vi "Read Track.vi"(7 "Track Controls":T1 {"Track 3"."Volume Settings"."Volume" scale=1.0..10.0; "Track 3"."Volume Settings"."Pan" scale=0.0..1.0; "Track 3"."Effects Settings"."Delay 2" scale=0.0..10.0; "Track 3"."Effects Settings"."Delay" scale=0.0..1.0; "Track 2"."Volume Settings"."Volume" scale=1.0..10.0; "Track 2"."Volume Settings"."Pan" scale=0.0..1.0; "Track 2"."Effects Settings"."Delay 2" scale=0.0..10.0; "Track 2"."Effects Settings"."Delay" scale=0.0..1.0; "Track 1"."Volume Settings"."Volume" scale=1.0..10.0; "Track 1"."Volume Settings"."Pan" scale=0.0..1.0; "Track 1"."Effects Settings"."Delay 2" scale=0.0..10.0; "Track 1"."Effects Settings"."Delay" scale=0.0..1.0; "Track 0"."Volume Settings"."Volume" scale=1.0..10.0; "Track 0"."Volume Settings"."Pan" scale=0.0..1.0; "Track 0"."Effects Settings"."Delay 2" scale=0.0..10.0; "Track 0"."Effects Settings"."Delay" scale=0.0..1.0}, 8 "Error In":errorcluster, 9 "Number Of Elements to Read":i64, 10 "Read Position":i64, 11 "Track (File) References In":T5) -> (0 "Error Out":errorcluster, 2 "4-Track Audio":T6, 3 "Track (File) References Out":T5)   [LabVIEW 2014]
doc: "Use this VI to read audio data from Tracks. This function will always read and return both Left and Right channels. You must provide the VI with:\n\nTrack File References: Track Ref + Track Name. \nRead Position: Specifies where to start reading from.\nNumber of Elements: Specifies how many elements to read. \nTrack Enable: Define which tracks you want to read. Setting to True will enables reading from the track. \nChannel Write Positions: Can specify a starting\\offset write position for each track you want to write too."
uses:
  Controls/4 Track Audio.ctl
  Controls/Audio In.ctl
  Controls/Track (File) References.ctl
  Controls/Track Controls.ctl
  Controls/Track Settings.ctl
  Controls/Track Effects Settings.ctl
  Controls/Track Volume Settings.ctl
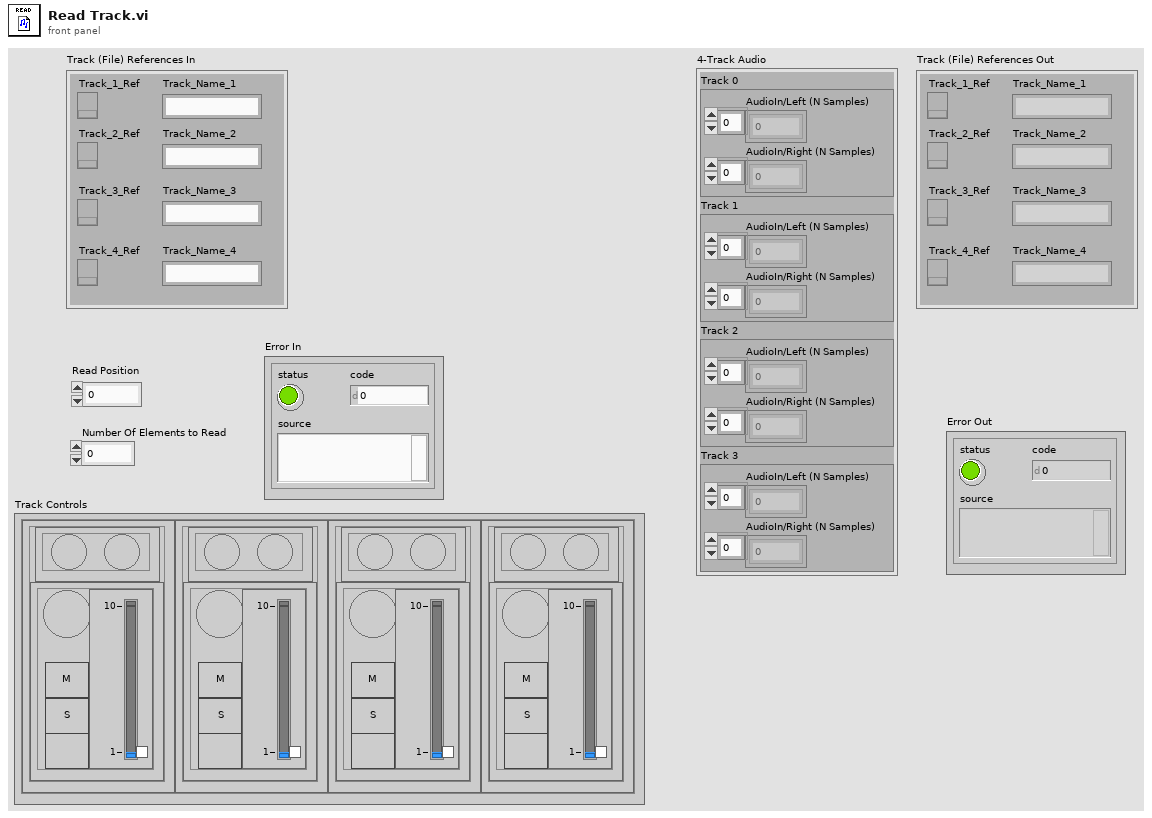
[diagram p1: front panel]
types:
  T1 = typedef "Track Controls.ctl" = cluster{"Track 0":T2, "Track 1":T2, "Track 2":T2, "Track 3":T2}
  T2 = typedef "Track Settings.ctl" = cluster{"Effects Settings":T3, "Volume Settings":T4}
  T3 = typedef "Track Effects Settings.ctl" = cluster{"Delay":dbl, "Delay 2":dbl}
  T4 = typedef "Track Volume Settings.ctl" = cluster{"Mute":bool, "Solo":bool, "Record":bool, "Pan":dbl, "Volume":dbl}
  T5 = typedef "Track (File) References.ctl" = cluster{"Track_1_Ref":refnum<k34>, "Track_2_Ref":refnum<k34>, "Track_3_Ref":refnum<k34>, "Track_4_Ref":refnum<k34>, "Track_Name_1":string, "Track_Name_2":string, "Track_Name_3":string, "Track_Name_4":string}
  T6 = typedef "4 Track Audio.ctl" = cluster{"Track 0":T7, "Track 1":T7, "Track 2":T7, "Track 3":T7}
  T7 = typedef "Audio In.ctl" = cluster{"AudioIn/Left (N Samples)":i16[], "AudioIn/Right (N Samples)":i16[]}
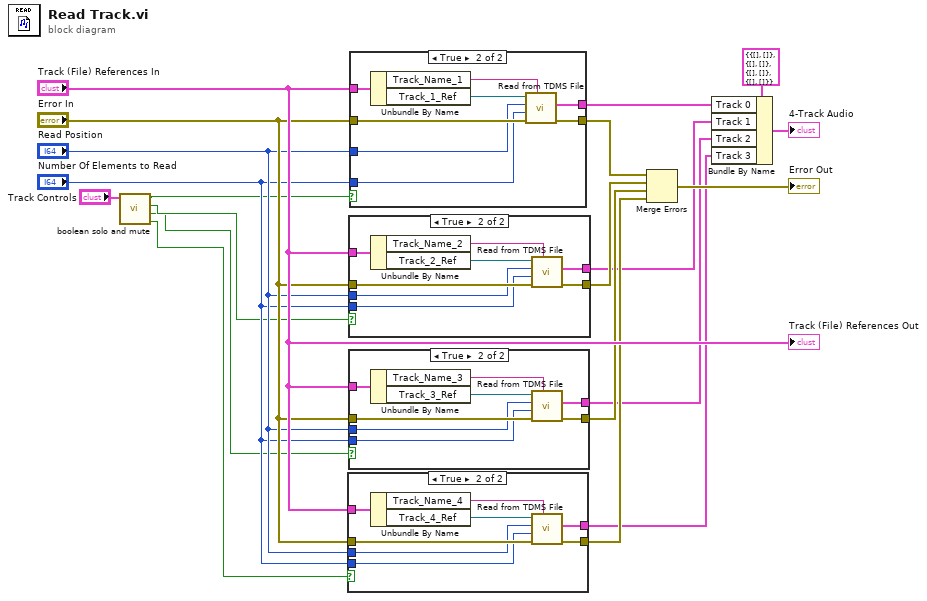
[diagram p0: block diagram]
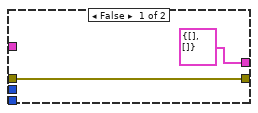
[diagram p2: hidden frame]
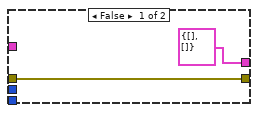
[diagram p3: hidden frame]
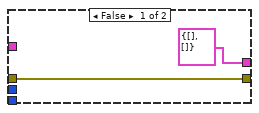
[diagram p4: hidden frame]
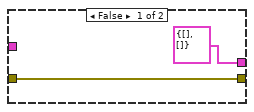
[diagram p5: hidden frame]
diagram:
  n1 = call "boolean solo and mute.vi"("Track Controls"="Track Controls") -> ("Track 3"=w2:bool, "Track 2"=w3:bool, "Track 1"=w4:bool, "Track 0"=w5:bool)  [unwired: 7 in]
  n2 = case shown="True" w2 {
    tunnel: "Track (File) References In" -> [_ w30]
    tunnel: "Error In" -> [w22 w27]
    tunnel: "Number Of Elements to Read" -> [_ w25]
    tunnel: "Read Position" -> [_ w26]
    tunnel: [w22 w24] -> w12
    tunnel: [T7 {"AudioIn/Left (N Samples)"=[], "AudioIn/Right (N Samples)"=[]} ("Audio Out") w23] -> w7
    frame False {
    }
    frame True {
      n3 = Unbundle By Name(w30) -> ("Track_Name_4"=w29:string, "Track_4_Ref"=w28:refnum<k34>)
      n4 = call "Read from TDMS File.vi"("Track Name"=w29, "Error In"=w27, "Number of Elements"=w25, "Read Position"=w26, "TDMS Reference In"=w28) -> ("Error Out"=w24:errorcluster, "Audio Out"=w23:T7)  [unwired: 4 in, 1 out]
    }
  }
  n5 = case shown="True" w4 {
    tunnel: "Track (File) References In" -> [_ w40]
    tunnel: "Error In" -> [w32 w37]
    tunnel: "Number Of Elements to Read" -> [_ w35]
    tunnel: "Read Position" -> [_ w36]
    tunnel: [w32 w34] -> w18
    tunnel: [T7 {"AudioIn/Left (N Samples)"=[], "AudioIn/Right (N Samples)"=[]} ("Audio Out") w33] -> w6
    frame False {
    }
    frame True {
      n6 = Unbundle By Name(w40) -> ("Track_Name_2"=w39:string, "Track_2_Ref"=w38:refnum<k34>)
      n7 = call "Read from TDMS File.vi"("Track Name"=w39, "Error In"=w37, "Number of Elements"=w35, "Read Position"=w36, "TDMS Reference In"=w38) -> ("Error Out"=w34:errorcluster, "Audio Out"=w33:T7)  [unwired: 4 in, 1 out]
    }
  }
  n8 = case shown="True" w3 {
    tunnel: "Track (File) References In" -> [_ w50]
    tunnel: "Error In" -> [w42 w47]
    tunnel: "Number Of Elements to Read" -> [_ w45]
    tunnel: "Read Position" -> [_ w46]
    tunnel: [w42 w44] -> w13
    tunnel: [T7 {"AudioIn/Left (N Samples)"=[], "AudioIn/Right (N Samples)"=[]} ("Audio Out") w43] -> w8
    frame False {
    }
    frame True {
      n9 = Unbundle By Name(w50) -> ("Track_Name_3"=w49:string, "Track_3_Ref"=w48:refnum<k34>)
      n10 = call "Read from TDMS File.vi"("Track Name"=w49, "Error In"=w47, "Number of Elements"=w45, "Read Position"=w46, "TDMS Reference In"=w48) -> ("Error Out"=w44:errorcluster, "Audio Out"=w43:T7)  [unwired: 4 in, 1 out]
    }
  }
  n11 = case shown="True" w5 {
    tunnel: "Track (File) References In" -> [_ w60]
    tunnel: "Error In" -> [w52 w57]
    tunnel: "Number Of Elements to Read" -> [_ w55]
    tunnel: "Read Position" -> [_ w56]
    tunnel: [w52 w54] -> w19
    tunnel: [T7 {"AudioIn/Left (N Samples)"=[], "AudioIn/Right (N Samples)"=[]} ("Audio Out") w53] -> w9
    frame False {
    }
    frame True {
      n12 = Unbundle By Name(w60) -> ("Track_Name_1"=w59:string, "Track_1_Ref"=w58:refnum<k34>)
      n13 = call "Read from TDMS File.vi"("Track Name"=w59, "Error In"=w57, "Number of Elements"=w55, "Read Position"=w56, "TDMS Reference In"=w58) -> ("Error Out"=w54:errorcluster, "Audio Out"=w53:T7)  [unwired: 4 in, 1 out]
    }
  }
  n14 = Merge Errors(w19, w18, w13, w12) -> (→"Error Out":errorcluster)
  n15 = Bundle By Name(cluster=T6 {"Track 0"={"AudioIn/Left (N Samples)"=[], "AudioIn/Right (N Samples)"=[]}, "Track 1"={"AudioIn/Left (N Samples)"=[], "AudioIn/Right (N Samples)"=[]}, "Track 2"={"AudioIn/Left (N Samples)"=[], "AudioIn/Right (N Samples)"=[]}, "Track 3"={"AudioIn/Left (N Samples)"=[], "AudioIn/Right (N Samples)"=[]}} ("4-Track Audio"), "Track 0"=w9, "Track 1"=w6, "Track 2"=w8, "Track 3"=w7) -> (→"4-Track Audio":T6)
  "Track (File) References Out" <- "Track (File) References In"
